vi "SendConfig API.vi"(8 "Error In":errorcluster) -> (0 "Error Out":errorcluster)   [LabVIEW 2017, in "Auto cycle.lvlib"]
uses:
  Auto cycle.lvlib
  Monochromator/Controls/Command Data [cluster].ctl
  Monochromator/Controls/Commands [enum].ctl
  Monochromator/Controls/Params.ctl
  Monochromator/Controls/Type.ctl
  Monochromator/Controls/GratingValues.ctl
  Monochromator/Controls/Grating.ctl
  Monochromator/PTI/Controls/Params.ctl
  Monochromator/Controls/VISA parameters.ctl
  Monochromator/Custom Oriel drivers/Controls/Params.ctl
  Monochromator/Oriel/Controls/Params.ctl
  C:/Project Work/icl-optical-software-rewrite/Optical Software Code Simplified/Modules/Monochromator/Cornerstone.dll
  Monochromator/Cornerstone.dll
  Events/Events.lvlib
  Monochromator/Monochromator.lvlib
  Serial comms/Serial comms.lvlib
  Monochromator/Oriel/Oriel (old drivers).lvlib
  Monochromator/Custom Oriel drivers/Oriel (custom drivers).lvlib
  Monochromator/PTI/PTI.lvlib
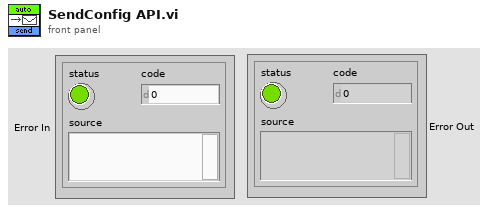
[diagram p1: front panel]
types:
  T1 = typedef "Monochromator.lvlib/Params.ctl" = cluster{"Type":T2, "Wavelength (nm)":dbl, "Grating, gr/mm":T3, "Grating mode":T4, "Spectrum mode":cluster{"Spectrum mode?":bool, "Start wavelength (nm)":dbl, "End wavelength (nm)":dbl, "Wavelength step (nm)":dbl, "Wavelength array":dbl[], "array index":u32}, "PTI":T5, "Oriel (custom)":T7, "Oriel (old)":T8, "Force wavelength confirmation (PTI)?":bool}
  T2 = typedef "Monochromator.lvlib/Type.ctl" = enum32{"Oriel", "PTI"}
  T3 = typedef "Monochromator.lvlib/GratingValues.ctl" = enum16{"2400", "1800", "1200", "600", "300", "150"}
  T4 = typedef "Monochromator.lvlib/Grating.ctl" = enum32{"unknown", "Visible", "IR"}
  T5 = typedef "Monochromator.lvlib/PTI.lvlib/Params.ctl" = cluster{"delay before read (ms)":u32, "Mono 1":T6, "Mono 2":T6}
  T6 = typedef "Serial comms.lvlib/VISA parameters.ctl" = cluster{"Enable Termination Char (T)":bool, "timeout (ms)":u32, "Resource name":refnum<visa-resource-name>, "baud rate":u32, "data bits":u16, "parity":u16, "stop bits":u16, "flow control":u16}
  T7 = typedef "Monochromator.lvlib/Oriel (custom drivers).lvlib/Params.ctl" = cluster{"reference":refnum<k24>}
  T8 = typedef "Monochromator.lvlib/Oriel (old drivers).lvlib/Params.ctl" = cluster{"configuration file path":path}
  T9 = typedef "Monochromator.lvlib/Command Data [cluster].ctl" = cluster{"Command":T10, "Data":variant}
  T10 = typedef "Monochromator.lvlib/Commands [enum].ctl" = enum16{"Start", "Spectrum setup", "Spectrum move", "Monochromator Setup", "Move", "GetPosition", "Stop", "Send data"}
  T11 = typedef "Events.lvlib/Refs [cluster].ctl" = cluster{"Exit":refnum<user-event>, "Controller":refnum<user-event>, "System Error":refnum<user-event>, "UI":refnum<user-event>, "Example Module":refnum<user-event>, "Shutter":refnum<user-event>, "Monochromator":refnum<user-event>, "DAQ":refnum<user-event>, "Scope":refnum<user-event>, "Auto cycle":refnum<user-event>, "Processing":refnum<user-event>, "File IO":refnum<user-event>, "Colour wheel":refnum<user-event>}
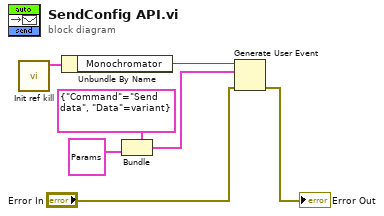
[diagram p0: block diagram]
diagram:
  n1 = call "Init ref kill.vi"() -> ("Messages"=w7:T11)  [unwired: 10 in, 1 out]
  n2 = Unbundle By Name(w7) -> ("Monochromator"=w6:refnum<user-event>)
  n3 = Bundle(cluster=T9 {"Command"=enum."Send data", "Data"=variant} ("event data"), "Data"=T1 {"Type"=enum."PTI", "Wavelength (nm)"=600.0, "Grating, gr/mm"=enum."1200", "Grating mode"=enum."unknown", "Spectrum mode"={"Spectrum mode?"=FALSE, "Start wavelength (nm)"=0.0, "End wavelength (nm)"=0.0, "Wavelength step (nm)"=0.0, "Wavelength array"=[], "array index"=0}, "PTI"={"delay before read (ms)"=50, "Mono 1"={"Enable Termination Char (T)"=FALSE, "timeout (ms)"=1000, "Resource name"="COM1", "baud rate"=9600, "data bits"=8, "parity"=0, "stop bits"=10, "flow control"=0}, "Mono 2"={"Enable Termination Char (T)"=FALSE, "timeout (ms)"=1000, "Resource name"="COM1", "baud rate"=9600, "data bits"=8, "parity"=0, "stop bits"=10, "flow control"=0}}, "Oriel (custom)"={"reference"=refnum}, "Oriel (old)"={"configuration file path"=path ""}, "Force wavelength confirmation (PTI)?"=FALSE} ("Monochromator")) -> (w4:T9)  [unwired: 1 in]
  n4 = Generate User Event(user event=w6, event data cluster=w4, error in="Error In") -> (error out=→"Error Out":errorcluster)  [unwired: 1 in, 1 out]
